vi "Automatic DATA File Select (SubVI).vi"(11 "name or relative path":path) -> (3 "actual path":path)   [LabVIEW 2020]
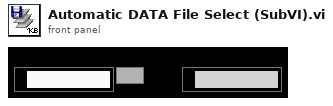
[diagram p1: front panel]
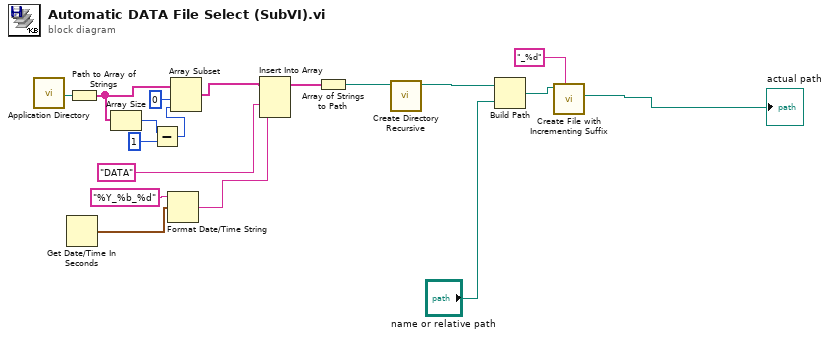
[diagram p0: block diagram]
diagram:
  n1 = call <vilib>:"Application Directory.vi"() -> ("Application Directory"=w3:path)
  n2 = Get Date/Time In Seconds() -> (seconds since 1Jan1904=w2:timestamp)
  n3 = Path to Array of Strings(0:w3) -> (2:w8:string[])  [unwired: 1 out]
  n4 = Array Size(array=w8) -> (size(s)=w5:i32)
  n5 = Subtract(x=w5, y=1) -> (x-y=w7:i32)
  n6 = Format Date/Time String(time format string (%c)="%Y_%b_%d", seconds (now)=w2) -> (date/time string=w11:string)  [unwired: 1 in]
  n7 = Array Subset(array=w8, index=0, length=w7) -> (w9:string[])
  n8 = Insert Into Array(array=w9, new element #1="DATA", new element #2=w11) -> (w12:string[])  [unwired: 1 in]
  n9 = Array of Strings to Path(0:w12) -> (2:w13:path)  [unwired: 1 in]
  n10 = call <vilib>:"Create Directory Recursive.vi"("directory"=w13) -> ("directory copy"=w15:path)  [unwired: 4 in, 2 out]
  n11 = Build Path(base path=w15, name or relative path="name or relative path") -> (appended path=w16:path)
  n12 = call <vilib>:"Create File with Incrementing Suffix.vi"("format string (\" (%d)\")"="_%d" ("format string (\" (%d)\")"), "file path"=w16) -> ("actual path"=→"actual path":path)  [unwired: 7 in, 2 out]
